vi "Tree selection apply locks.vi"(8 "error in (no error)":errorcluster, 10 "Lock States":bool[](array[boolean]), 11 "Loop data":T1) -> (0 "error out":errorcluster, 3 "Loop data":T1)   [LabVIEW 2020, in "UI_ItemSelect.lvlib"]
uses:
  UI_ItemSelect.lvlib
  Tree item select loop data.ctl
  Item select ref type.ctl
  Tree item loop data.ctl
  Tree item selection indices.ctl
  checkbox state.ctl
  item select tree lock states.ctl
  <userlib>/Blue Origin/DeferPanelUpdates_OpenSource/SubVIs/defer panel updates Controlref step1.vi
  <userlib>/_OpenG.lib/array/array.llb/Index 1D Array Elements (Boolean)__ogtk.vi
  <userlib>/Blue Origin/DeferPanelUpdates_OpenSource/SubVIs/defer panel updates step2.vi
  <userlib>/Blue Origin/DeferPanelUpdates_OpenSource/Defer Panel Updates OpenSource.lvlib
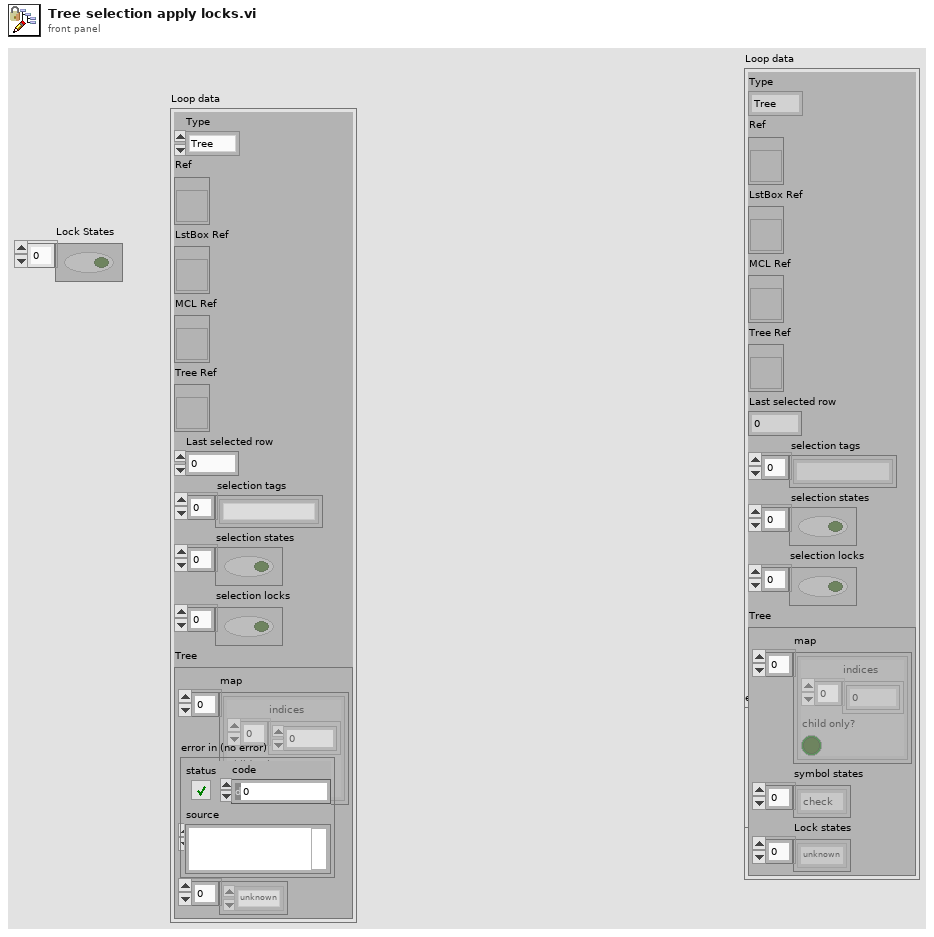
[diagram p1: front panel]
types:
  T1 = typedef "UI_ItemSelect.lvlib/Tree item select loop data.ctl" = cluster{"Type":T2, "Ref":refnum<vi>, "LstBox Ref":refnum<vi>, "MCL Ref":refnum<vi>, "Tree Ref":refnum<vi>, "Last selected row":i32, "selection tags":string[], "selection states":bool[], "selection locks":bool[], "Tree":T3}
  T2 = typedef "UI_ItemSelect.lvlib/Item select ref type.ctl" = enum16{"Tree", "MCL", "ListBox"}
  T3 = typedef "UI_ItemSelect.lvlib/Tree item loop data.ctl" = cluster{"map":T4[], "symbol states":T5[], "Lock states":T6[]}
  T4 = typedef "UI_ItemSelect.lvlib/Tree item selection indices.ctl" = cluster{"indices":i32[], "child only?":bool}
  T5 = typedef "UI_ItemSelect.lvlib/checkbox state.ctl" = enum16{"unknown", "check", "some", "no check"}
  T6 = typedef "UI_ItemSelect.lvlib/item select tree lock states.ctl" = enum16{"unknown", "locked", "unlocked"}
  T7 = typedef "Defer Panel Updates OpenSource.lvlib/defer panel updates data.ctl" = cluster{"Owning VI":refnum<vi>, "Front Panel":refnum<vi>, "performed?":bool}
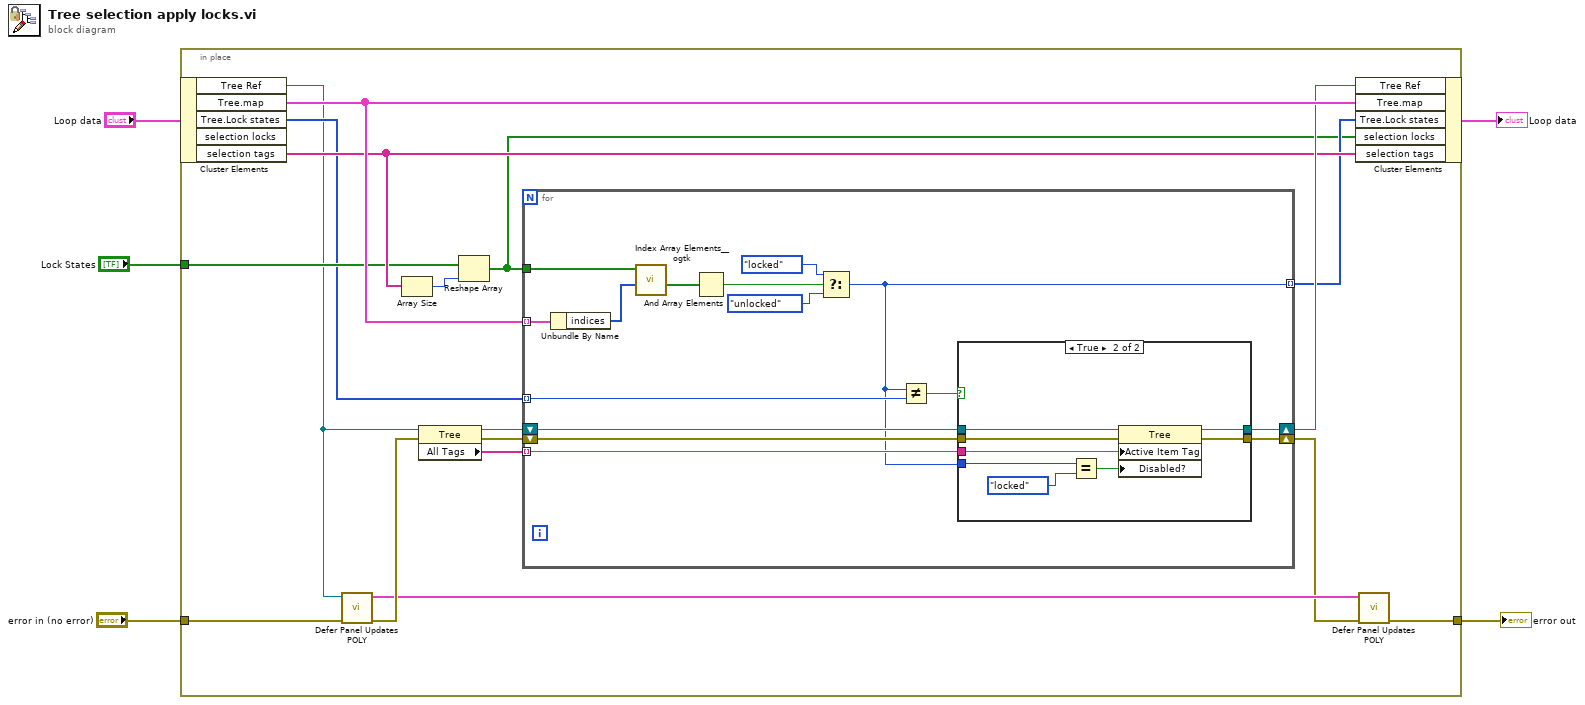
[diagram p0: block diagram]
diagram:
  n1 = in-place {
    in-place-border: "error in (no error)" -> [w11]
    in-place-border: [w6] -> w2
    in-place-border: "Lock States" -> [w15]
    n2 = in-place-cluster #1("Loop data") -> ("Tree Ref"=w10:refnum<vi>, "Tree.map"=w22:T4[], "Tree.Lock states"=w14:T6[], "selection tags"=w17:string[])  [unwired: 1 out]
    n3 = call-poly <userlib>:"Defer Panel Updates POLY.vi"("error in (no error)"=w11, "control reference"=w10) -> ("error out"=w9:errorcluster, "Refs"=w8:T7)  [unwired: 8 in]
    n4 = Array Size(array=w17) -> (size(s)=w16:i32)
    n5 = property class="Tree"(reference=w10, error in=w9) -> (reference out=w21:refnum<vi>, error out=w19:errorcluster, "All Tags"=w20:string[])
    n6 = Reshape Array(w15, w16) -> (w12:bool[])
    n7 = for {
      tunnel: w22 -> [w37] mode=indexing
      tunnel: w12 -> [w36]
      tunnel: [w23] -> w13 mode=indexing
      tunnel: w14 -> [w31] mode=indexing
      tunnel: w20 -> [w32] mode=indexing
      shift-right: [w28] -> w7
      shift-left: w19 -> [w29]
      shift-right: [w27] -> w18
      shift-left: w21 -> [w33]
      n8 = Unbundle By Name(w37) -> ("indices"=w35:i32[])
      n9 = call-poly <userlib>:"Index Array Elements__ogtk.vi"("indices"=w35, "array"=w36) -> ("elements"=w34:bool[])  [unwired: 9 in]
      n10 = And Array Elements(Boolean array=w34) -> (logical AND=w26:bool)
      n11 = Select(t=item_select_tree_lock_states."locked" ("Enum"), s=w26, f=item_select_tree_lock_states."unlocked" ("Enum")) -> (s? t:f=w23:T6)
      n12 = Not Equal?(x=w23, y=w31) -> (x != y?=w30:bool)
      n13 = case shown="True" w30 {
        tunnel: w33 -> [w38 w47]
        tunnel: w32 -> [_ w46]
        tunnel: w23 -> [_ w42]
        tunnel: w29 -> [w39 w45]
        tunnel: [w39 w44] -> w28
        tunnel: [w38 w43] -> w27
        frame False {
        }
        frame True {
          n14 = Equal?(x=w42, y=item_select_tree_lock_states."locked" ("Enum")) -> (x = y?=w41:bool)
          n15 = property class="Tree"(reference=w47, error in=w45, "Active Item Tag"=w46, "Disabled?"=w41) -> (reference out=w43:refnum<vi>, error out=w44:errorcluster)
        }
      }
    }
    n16 = in-place-cluster #1("Tree Ref"=w18, "Tree.map"=w22, "Tree.Lock states"=w13, "selection locks"=w12, "selection tags"=w17) -> (→"Loop data":T1)
    n17 = call-poly <userlib>:"Defer Panel Updates POLY.vi"("error in (no error)"=w7, "Refs"=w8) -> ("error out"=w6:errorcluster)  [unwired: 9 in]
  }
  "error out" <- w2
